vi "Get Path to UI Subpanel.vi"(8 "error in (no error)":errorcluster, 10 "Calling VI":refnum<vi>, 11 "packed library path":path=path "C:/Users/Public/Documents/CIF/PluginUI/CIF Template UI.2.0.0.lvlibp") -> (0 "error out":errorcluster, 3 "Path to Subpanel":path)   [LabVIEW 2021, in "CIF_UI.lvclass"]
uses:
  CIF_UI.lvclass
  <vilib>/Utility/LVLibp/NI_PackedLibraryUtility.lvlib
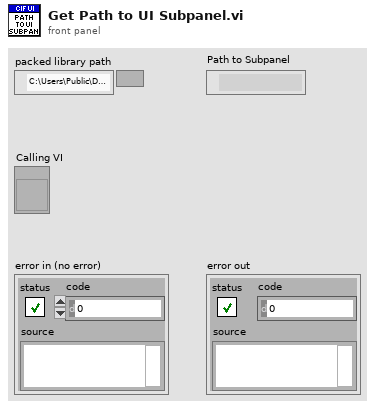
[diagram p1: front panel]
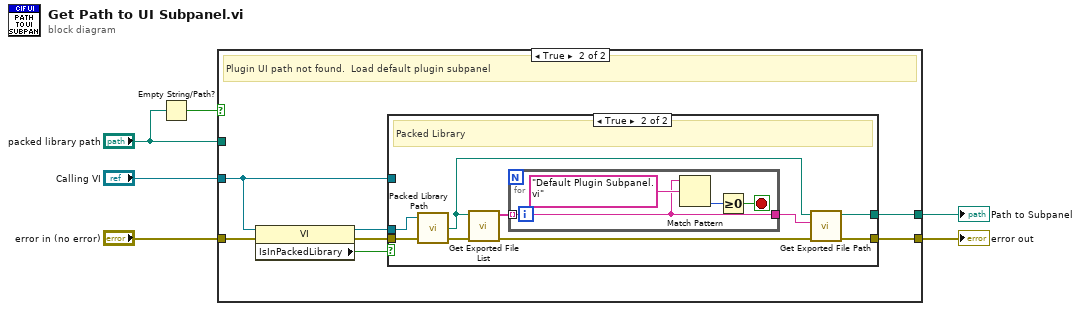
[diagram p0: block diagram]
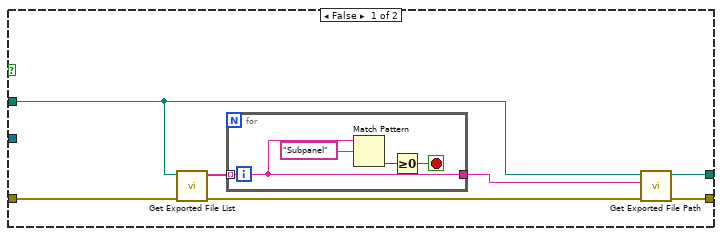
[diagram p2: hidden frame]
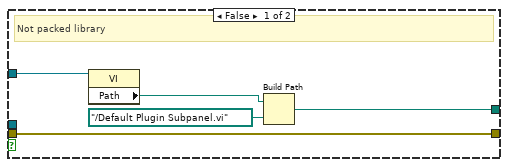
[diagram p3: hidden frame]
diagram:
  n1 = Empty String/Path?(string/path="packed library path") -> (empty?=w2:bool)
  n2 = case shown="True" w2 {
    tunnel: "error in (no error)" -> [w10 w21]
    tunnel: [w9 w20] -> w5
    tunnel: [w8 w19] -> w4
    tunnel: "packed library path" -> [w7 _]
    tunnel: "Calling VI" -> [_ w18]
    frame False {
      n3 = call <vilib>:"Get Exported File List.vi"("error in (no error)"=w10, "packed library path"=w7) -> ("error out"=w12:errorcluster, "qualified names"=w13:string[])  [unwired: 7 in, 1 out]
      n4 = for {
        tunnel: w13 -> [w14] mode=indexing
        tunnel: [w14] -> w11
        stop <- w16 stop-if-true
        n5 = Match Pattern(string=w14, regular expression="Subpanel") -> (offset past match=w17:i32)  [unwired: 1 in, 3 out]
        n6 = Greater Or Equal To 0?(x=w17) -> (x >= 0?=w16:bool)
      }
      n7 = call <vilib>:"Get Exported File Path.vi"("error in (no error)"=w12, "qualified name"=w11, "packed library path"=w7) -> ("error out"=w9:errorcluster, "path"=w8:path)  [unwired: 7 in]
    }
    frame True {
      # "Plugin UI path not found.  Load default plugin subpanel"
      n8 = property class="VI"(reference=w18, error in=w21) -> (reference out=w23:refnum<vi>, error out=w22:errorcluster, "IsInPackedLibrary"=w24:bool)
      n9 = case shown="True" w24 {
        tunnel: w23 -> [_ w38]
        tunnel: w22 -> [w27 w37]
        tunnel: [w29 w31] -> w19
        tunnel: [w27 w30] -> w20
        tunnel: w18 -> [w26 _]
        frame False {
          # "Not packed library"
          n10 = property class="VI"(reference=w26) -> ("Path"=w25:path)  [unwired: 1 in, 2 out]
          n11 = Build Path(base path=w25, name or relative path=path "../Default Plugin Subpanel.vi" ("Path")) -> (appended path=w29:path)
        }
        frame True {
          # "Packed Library"
          n12 = call <vilib>:"Packed Library Path.vi"("error in (no error)"=w37, "vi reference"=w38) -> ("error out"=w32:errorcluster, "packed library path"=w33:path)  [unwired: 1 in, 1 out]
          n13 = call <vilib>:"Get Exported File List.vi"("error in (no error)"=w32, "packed library path"=w33) -> ("error out"=w35:errorcluster, "qualified names"=w34:string[])  [unwired: 7 in, 1 out]
          n14 = for {
            tunnel: w34 -> [w39] mode=indexing
            tunnel: [w39] -> w36
            stop <- w41 stop-if-true
            n15 = Match Pattern(string=w39, regular expression="Default Plugin Subpanel.vi") -> (offset past match=w42:i32)  [unwired: 1 in, 3 out]
            n16 = Greater Or Equal To 0?(x=w42) -> (x >= 0?=w41:bool)
          }
          n17 = call <vilib>:"Get Exported File Path.vi"("error in (no error)"=w35, "qualified name"=w36, "packed library path"=w33) -> ("error out"=w30:errorcluster, "path"=w31:path)  [unwired: 7 in]
        }
      }
    }
  }
  "error out" <- w5
  "Path to Subpanel" <- w4
